vi "To String Array.vi"(8 "error in (no error)":errorcluster, 11 "String Compare Config in":refnum<class "String Compare Config.lvclass">) -> (0 "error out":errorcluster, 1 "Step String Array":string[](array[string]), 3 "String Compare Config out":refnum<class "String Compare Config.lvclass">)   [LabVIEW 2015, in "String Compare Config.lvclass"]
uses:
  String Compare Config.lvclass
  String Compare Config.lvclass/String Compare Config.ctl
  <vilib>/NI/Tag Bus/tag/tag descriptor.lvclass/tag descriptor.ctl
  Read Test Value Channel.vi
  Read Result Channel.vi
  Read Mode.vi
  Read Limit_Regex.vi
  Read Ignore Case.vi
  Read Multiline.vi
  Read offset.vi
  classes/Step/Config/Step Config.lvclass
  <vilib>/NI/Tag Bus Module Framework/channel/TBM channel.lvclass
  <vilib>/NI/Tag Bus/tag/tag descriptor.lvclass
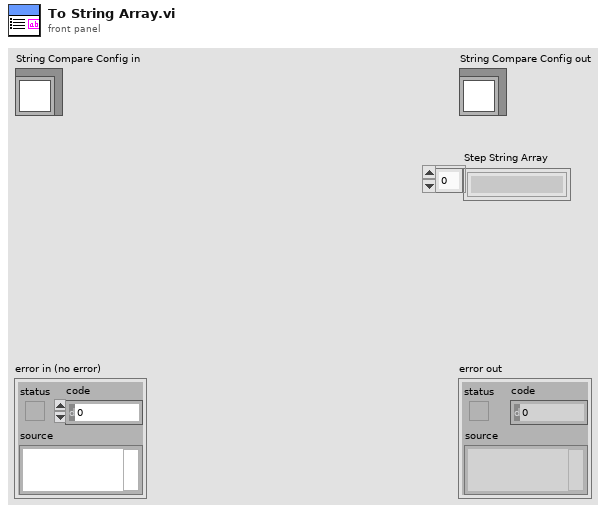
[diagram p1: front panel]
types:
  T1 = typedef "Mode.ctl" = enum16{"Compare Strings", "Match Regex"}
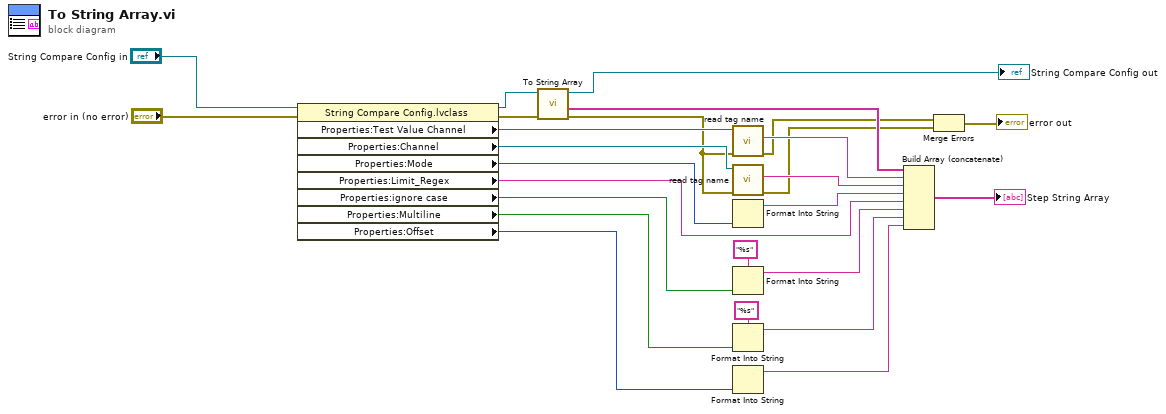
[diagram p0: block diagram]
diagram:
  n1 = property class="String Compare Config.lvclass"(reference="String Compare Config in", error in="error in (no error)") -> (reference out=w5:refnum<class "String Compare Config.lvclass">, error out=w2:errorcluster, "Properties:Test Value Channel"=w25:refnum<class "TBM channel.lvclass">, "Properties:Channel"=w24:refnum<class "TBM channel.lvclass">, "Properties:Mode"=w23:T1, "Properties:Limit_Regex"=w19:string, "Properties:ignore case"=w14:bool, "Properties:Multiline"=w13:bool, "Properties:Offset"=w12:i32)
  n2 = call-parent "To String Array.vi"("error in (no error)"=w2, "Step Config in"=w5) -> ("error out"=w1:errorcluster, "Step String Array"=w26:string[], "Step Config out"=→"String Compare Config out":refnum<class "String Compare Config.lvclass">)  [unwired: 7 in]
  n3 = call <vilib>:"read tag name.vi"("error in"=w1, "system tag in"=w25) -> ("error out"=w9:errorcluster, "name"=w22:string)  [unwired: 7 in, 1 out]
  n4 = call <vilib>:"read tag name.vi"("error in"=w1, "system tag in"=w24) -> ("error out"=w8:errorcluster, "name"=w21:string)  [unwired: 7 in, 1 out]
  n5 = Format Into String(w23) -> (resulting string=w20:string)  [unwired: 3 in, 1 out]
  n6 = Format Into String(format string="%s", w14) -> (resulting string=w17:string)  [unwired: 2 in, 1 out]
  n7 = Format Into String(format string="%s", w13) -> (resulting string=w15:string)  [unwired: 2 in, 1 out]
  n8 = Format Into String(w12) -> (resulting string=w11:string)  [unwired: 3 in, 1 out]
  n9 = Build Array (concatenate)(w26, w22, w21, w20, w19, w17, w15, w11) -> (→"Step String Array":string[])
  n10 = Merge Errors(w9, w8) -> (→"error out":errorcluster)
